vi "_Error-FunctionNotAvailable.vi"() -> (0 "error out":errorcluster)   [LabVIEW 2014, in "hse-db.lvlib" / "DB-ADO.lvclass"]
uses:
  DB-ADO.lvclass
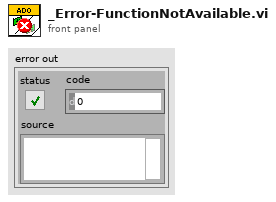
[diagram p1: front panel]
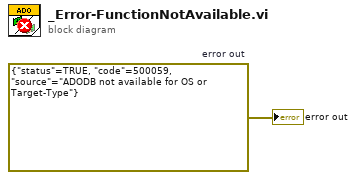
[diagram p0: block diagram]
diagram:
  w1 = errorcluster {"status"=TRUE, "code"=500059, "source"="ADODB not available for OS or Target-Type"}  # error out
  "error out" <- w1
